vi "rscmxpbase_FormatSIMSlotRepCapString_WriteCallback.vi"(5 "Attribute":T1={"Identifier"="", "Descriptive Name"="", "Data Type"=enum."Integer 32", "Command"="", "Access"=enum."Read/Write", "Range Table"="", "Read Callback"="", "Write Callback"="", "Supported Models"="", "Instrument Options"="", "Index"=0, "OPC Wait"=FALSE, "No Status Check"=FALSE, "Cache Only"=FALSE}, 7 "Repeated Capability":string, 8 "error in (no error)":errorcluster, 10 "Attribute Value String":string, 11 "VISA resource name":refnum<visa-resource-name>) -> (0 "error out":errorcluster, 3 "VISA resource name out":refnum<visa-resource-name>)   [LabVIEW 2020, in "Rohde&Schwarz CMXP Base.lvlib"]
doc: "Replaces <SIMSlot> with the value of the RSCMXPBASE_ATTR_SELECT_DUT_SIM_SLOT attribute."
uses:
  <instrlib>/Rohde&Schwarz CMXP Base/Rohde&Schwarz CMXP Base.lvlib
  <instrlib>/Rohde&Schwarz CMXP Base/Private/rsidr_core.llb/type_Attribute.ctl
  <instrlib>/Rohde&Schwarz CMXP Base/Private/rsidr_core.llb/type_Attribute_Data_Type.ctl
  <instrlib>/Rohde&Schwarz CMXP Base/Private/rsidr_core.llb/type_ReadWriteAccess.ctl
  <instrlib>/Rohde&Schwarz CMXP Base/Private/rsidr_core.llb/rsidr_core.lvlib
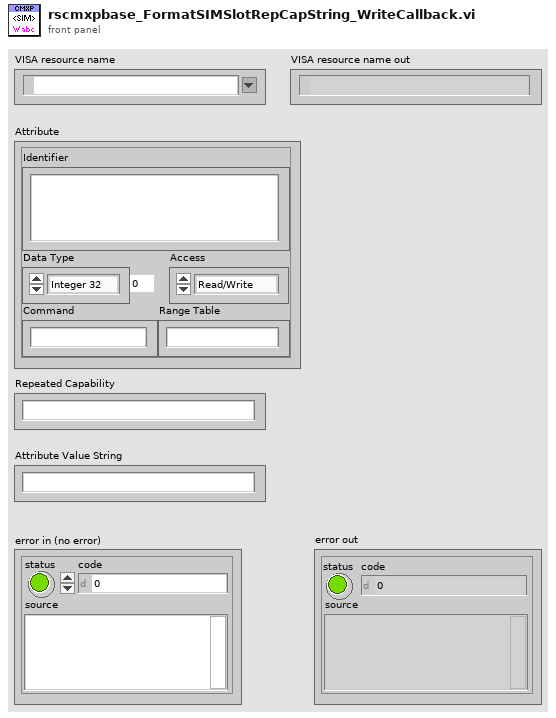
[diagram p1: front panel]
types:
  T1 = typedef "Rohde&Schwarz CMXP Base.lvlib/rsidr_core.lvlib/type_Attribute.ctl" = cluster{"Identifier":string, "Descriptive Name":string, "Data Type":T2, "Command":string, "Access":T3, "Range Table":string, "Read Callback":string, "Write Callback":string, "Supported Models":string, "Instrument Options":string, "Index":i32, "OPC Wait":bool, "No Status Check":bool, "Cache Only":bool}
  T2 = typedef "Rohde&Schwarz CMXP Base.lvlib/rsidr_core.lvlib/type_Attribute_Data_Type.ctl" = enum16{"Integer 32", "Double", "String", "Boolean", "None", "Integer 64", "RawString"}
  T3 = typedef "Rohde&Schwarz CMXP Base.lvlib/rsidr_core.lvlib/type_ReadWriteAccess.ctl" = enum16{"Read Only", "Write Only", "Read/Write"}
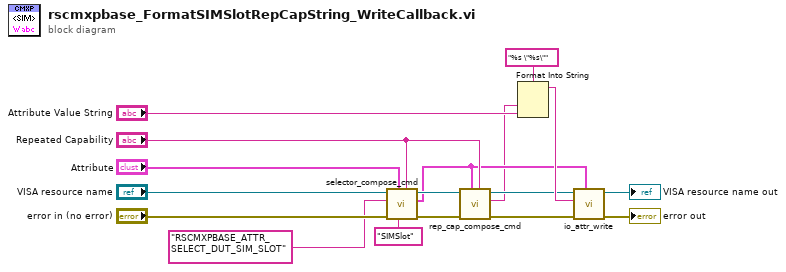
[diagram p0: block diagram]
diagram:
  n1 = call <instrlib>:"selector_compose_cmd.vi"("Repeated Capability"="Repeated Capability", "Selector Name"="SIMSlot", "Attribute"="Attribute", "error in"="error in (no error)", "Selector Attribute ID"="RSCMXPBASE_ATTR_SELECT_DUT_SIM_SLOT", "VISA resource name"="VISA resource name") -> ("error out"=w15:errorcluster, "Attribute out"=w5:T1, "VISA resource name out"=w10:refnum<visa-resource-name>)  [unwired: 3 in]
  n2 = call <instrlib>:"rep_cap_compose_cmd.vi"("Repeated Capability"="Repeated Capability", "Attribute"=w5, "error in"=w15, "VISA resource name"=w10) -> ("error out"=w3:errorcluster, "Command out"=w1:string, "VISA resource name out"=w4:refnum<visa-resource-name>)  [unwired: 5 in]
  n3 = Format Into String(format string="%s \"%s\"", w1, "Attribute Value String") -> (resulting string=w8:string)  [unwired: 2 in, 1 out]
  n4 = call <instrlib>:"io_attr_write.vi"("Attribute"=w5, "error in"=w3, "write buffer"=w8, "VISA resource name"=w4) -> ("error out"=→"error out":errorcluster, "VISA resource name out"=→"VISA resource name out":refnum<visa-resource-name>)  [unwired: 6 in]
